vi "GHV232 CRAB Query Response.vi"(10 "String":string) -> (0 "Fault":bool, 1 "HV on":bool, 2 "I mode":bool, 3 "V mode":bool, 4 "Current":dbl format="%#.2f", 5 "Voltage":dbl format="%#_2f", 6 "Checksum error":string)   [LabVIEW 2017]
panel:
  # "This VI decodes the 16 byte hexadecimal query response string.\nIt will display all analog and digital status monitors and give a \nchecksum error."
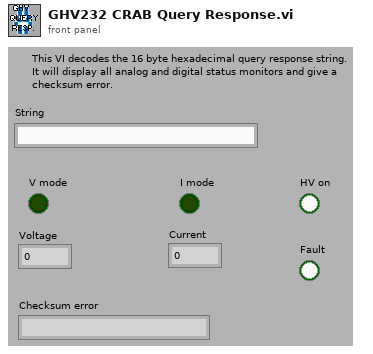
[diagram p1: front panel]
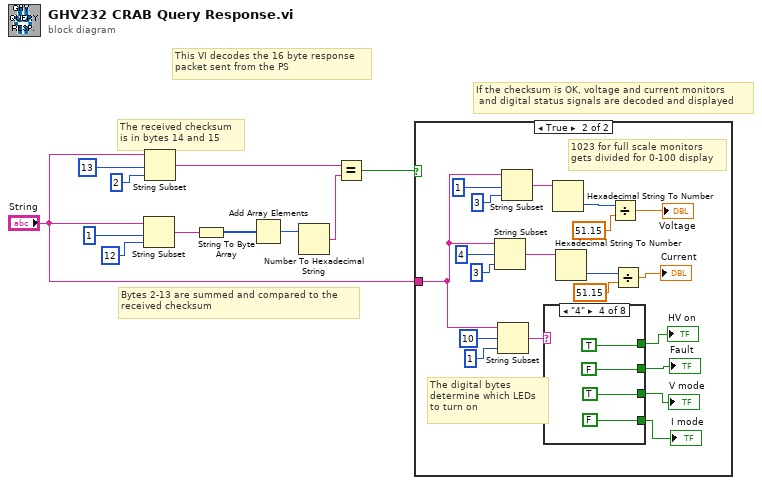
[diagram p0: block diagram]
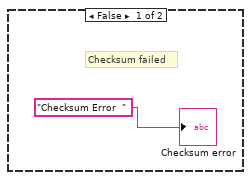
[diagram p2: hidden frame]
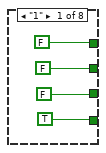
[diagram p3: hidden frame]
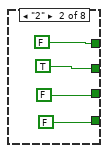
[diagram p4: hidden frame]
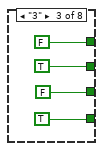
[diagram p5: hidden frame]
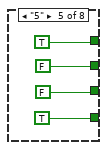
[diagram p6: hidden frame]
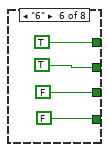
[diagram p7: hidden frame]
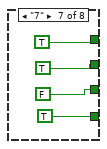
[diagram p8: hidden frame]
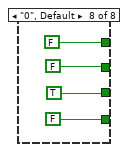
[diagram p9: hidden frame]
diagram:
  # "If the checksum is OK, voltage and current monitors\n and digital status signals are decoded and displayed"
  # "Bytes 2-13 are summed and compared to the\nreceived checksum"
  # "The received checksum\nis in bytes 14 and 15"
  # "This VI decodes the 16 byte response \npacket sent from the PS"
  n1 = String Subset(string="String", offset (0)=1, length (rest)=12) -> (substring=w3:string)
  n2 = String Subset(string="String", offset (0)=13, length (rest)=2) -> (substring=w5:string)
  n3 = String To Byte Array(string=w3) -> (unsigned byte array=w7:u8[])
  n4 = Add Array Elements(numeric array=w7) -> (sum=w6:u8)
  n5 = Number To Hexadecimal String(2:w6) -> (0:w2:string)  [unwired: 1 in]
  n6 = Equal?(x=w5, y=w2) -> (x = y?=w1:bool)
  n7 = case shown="True" w1 {
    tunnel: "String" -> [_ w26]
    frame False {
      # "Checksum failed"
      "Checksum error" <- "Checksum Error  "
    }
    frame True {
      # "The digital bytes\ndetermine which LEDs\nto turn on"
      # "1023 for full scale monitors\ngets divided for 0-100 display"
      n8 = String Subset(string=w26, offset (0)=4, length (rest)=3) -> (substring=w27:string)
      n9 = String Subset(string=w26, offset (0)=10, length (rest)=1) -> (substring=w14:string)
      n10 = String Subset(string=w26, offset (0)=1, length (rest)=3) -> (substring=w28:string)
      n11 = case shown="\"4\"" w14 {
        tunnel: [FALSE FALSE FALSE TRUE TRUE TRUE TRUE FALSE] -> w23
        tunnel: [FALSE TRUE TRUE FALSE FALSE TRUE TRUE FALSE] -> w22
        tunnel: [FALSE FALSE FALSE TRUE FALSE FALSE FALSE TRUE] -> w20
        tunnel: [TRUE FALSE TRUE FALSE TRUE FALSE TRUE FALSE] -> w21
        frame "1" {
        }
        frame "2" {
        }
        frame "3" {
        }
        frame "4" {
        }
        frame "5" {
        }
        frame "6" {
        }
        frame "7" {
        }
        frame "0", Default {
        }
      }
      "HV on" <- w23
      "Fault" <- w22
      "I mode" <- w21
      "V mode" <- w20
      n12 = Hexadecimal String To Number(string=w28) -> (number=w19:u32)  [unwired: 2 in, 1 out]
      n13 = Hexadecimal String To Number(string=w27) -> (number=w16:u32)  [unwired: 2 in, 1 out]
      n14 = Divide(x=w19, y=51.15) -> (x/y=→"Voltage":dbl)
      n15 = Divide(x=w16, y=51.15) -> (x/y=→"Current":dbl)
    }
  }
